vi "Opt2.vi"(0 "Activation Function":enum32{"Sigmoid", "RELU", "Tanh", "Leaky RELU"}(ring), 1 "Weights l+1":dbl[](array[numeric]), 2 "Weights":dbl[][](array[numeric]), 3 "Biases":dbl[](array[numeric]), 5 "Net Output":dbl[](array[numeric]), 7 "Activations l-1":dbl[](array[numeric]) format="%.2f", 9 "Delta l+1":dbl, 12 "Weight Regularizers":enum32{"None", "L1", "L2"}(radio), 13 "Adam Data In":T1) -> (4 "Delta l":dbl[](array[numeric]), 6 "Updated Weights":dbl[][](array[numeric]), 8 "Updated Biases":dbl[](array[numeric]), 14 "Adam Data Out":T1)   [LabVIEW 2018]
uses:
  Adam_data.ctl
  <vilib>/Analysis/baseanly.llb/Real Outer Product.vi
  <vilib>/Analysis/Matrix/Numeric/Conversions/Matrix To Array - RM.vi
  Iteration Counter.vi
  <vilib>/Analysis/NI_AALBase.lvlib
  <vilib>/Analysis/Matrix/NI_Matrix.lvlib
panel:
  out "Grad. w":dbl[][](array[numeric])
  out "Grad. b":dbl[](array[numeric])
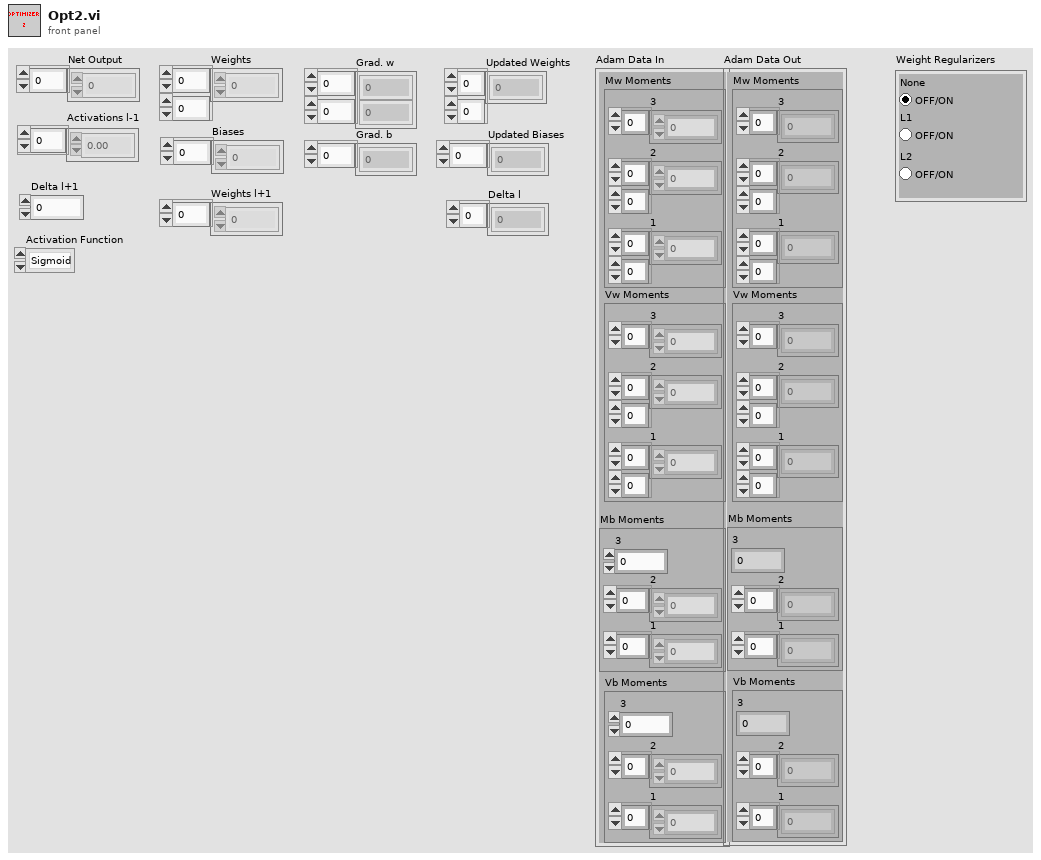
[diagram p1: front panel]
types:
  T1 = typedef "Adam_data.ctl" = cluster{"Mw Moments":cluster{"3 ":dbl[], "2":dbl[][], "1":dbl[][]}, "Vw Moments":cluster{"3":dbl[], "2":dbl[][], "1":dbl[][]}, "Mb Moments":cluster{"3":dbl, "2":dbl[], "1":dbl[]}, "Vb Moments":cluster{"3":dbl, "2":dbl[], "1":dbl[]}}
  T2 = typedef "NI_Matrix.lvlib/RealMatrix.ctl" = dbl[][]
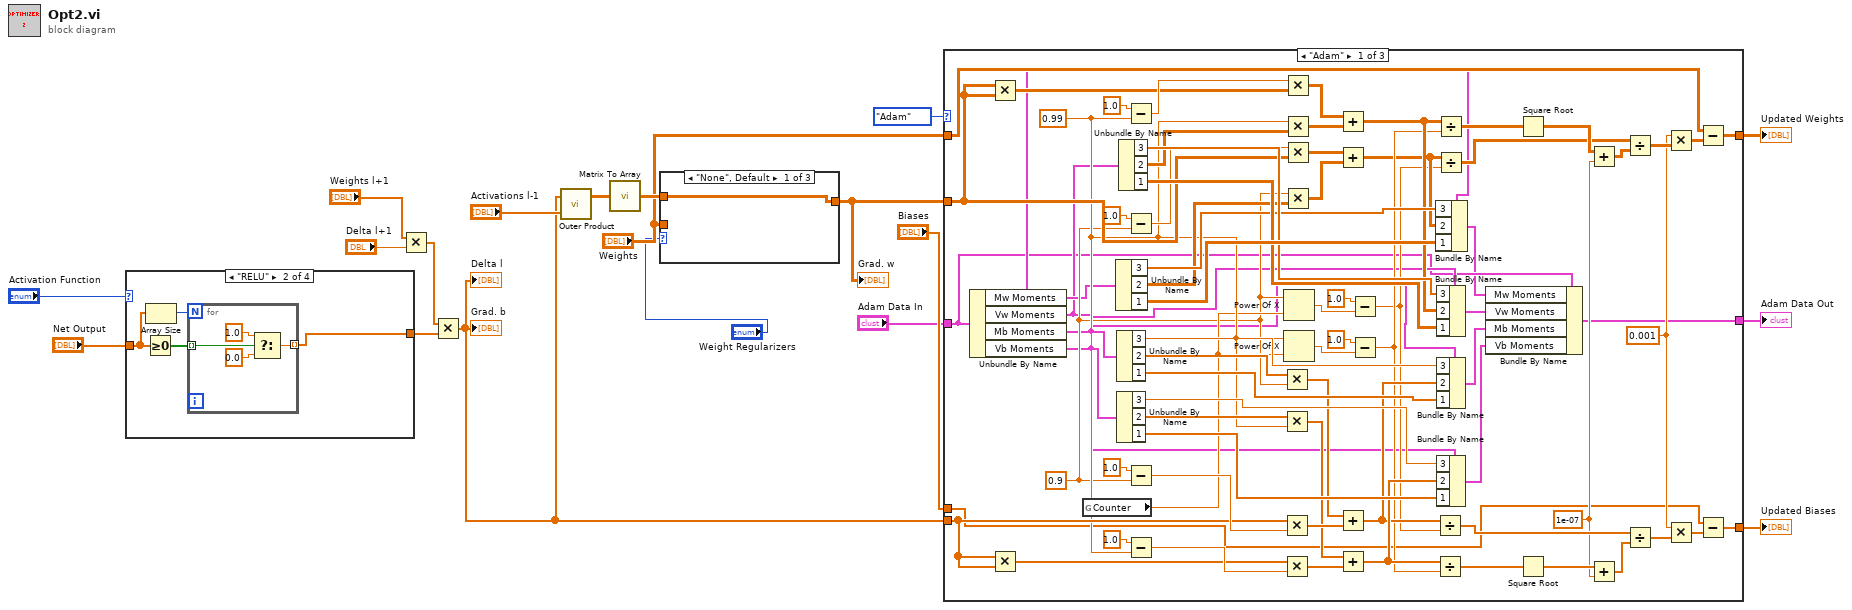
[diagram p0: block diagram]
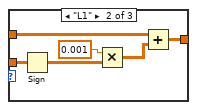
[diagram p2: hidden frame]
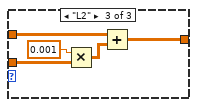
[diagram p3: hidden frame]
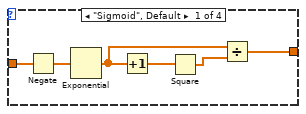
[diagram p6: hidden frame]
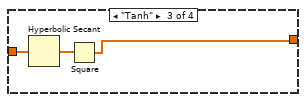
[diagram p7: hidden frame]
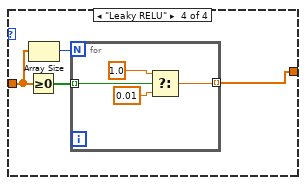
[diagram p8: hidden frame]
diagram:
  n1 = case shown="\"RELU\"" "Activation Function" {
    tunnel: "Net Output" -> [w21 w27 w35 w38]
    tunnel: [w20 w29 w34 w40] -> w18
    frame "Sigmoid", Default {
      n2 = Negate(x=w21) -> (-x=w25:dbl[])
      n3 = Exponential(1:w25) -> (0:w22:dbl[])
      n4 = Increment(x=w22) -> (x+1=w24:dbl[])
      n5 = Square(x=w24) -> (x^2=w23:dbl[])
      n6 = Divide(x=w22, y=w23) -> (x/y=w20:dbl[])
    }
    frame "RELU" {
      n7 = Greater Or Equal To 0?(x=w27) -> (x >= 0?=w28:bool[])
      n8 = Array Size(array=w27) -> (size(s)=w26:i32)
      n9 = for {
        N: w26 -> [_]
        tunnel: [w33] -> w29 mode=indexing
        tunnel: w28 -> [w30] mode=indexing
        n10 = Select(t=1.0, s=w30, f=0.0) -> (s? t:f=w33:dbl)
      }
    }
    frame "Tanh" {
      n11 = Hyperbolic Secant(1:w35) -> (0:w36:dbl[])
      n12 = Square(x=w36) -> (x^2=w34:dbl[])
    }
    frame "Leaky RELU" {
      n13 = Greater Or Equal To 0?(x=w38) -> (x >= 0?=w39:bool[])
      n14 = Array Size(array=w38) -> (size(s)=w37:i32)
      n15 = for {
        N: w37 -> [_]
        tunnel: [w42] -> w40 mode=indexing
        tunnel: w39 -> [w41] mode=indexing
        n16 = Select(t=1.0, s=w41, f=0.01) -> (s? t:f=w42:dbl)
      }
    }
  }
  n17 = Multiply(x="Weights l+1", y="Delta l+1") -> (x*y=w8:dbl[])
  n18 = Multiply(x=w8, y=w18) -> (x*y=w14:dbl[])
  "Grad. b" <- w14
  "Delta l" <- w14
  n19 = call-poly <vilib>:"Outer Product.vi"("Y Vector"="Activations l-1", "X Vector"=w14) -> ("Outer Product"=w13:T2)  [unwired: 1 out]
  n20 = call-poly <vilib>:"Matrix To Array.vi"("Real Matrix"=w13) -> ("Real 2D Array"=w4:dbl[][])
  n21 = case shown="\"None\", Default" "Weight Regularizers" {
    tunnel: w4 -> [w45 w47 w56]
    tunnel: [w45 w46 w52] -> w2
    tunnel: "Weights" -> [_ w50 w54]
    frame "None", Default {
    }
    frame "L1" {
      n22 = Sign(1:w50) -> (0:w49:dbl[][])
      n23 = Multiply(x=0.001, y=w49) -> (x*y=w48:dbl[][])
      n24 = Add(x=w47, y=w48) -> (x+y=w46:dbl[][])
    }
    frame "L2" {
      n25 = Multiply(x=0.001, y=w54) -> (x*y=w53:dbl[][])
      n26 = Add(x=w56, y=w53) -> (x+y=w52:dbl[][])
    }
  }
  "Grad. w" <- w2
  n27 = case shown="\"Adam\"" enum16{"Adagrad", "Adadelta", "Adam"}."Adam" ("Optimizer") {
    tunnel: "Weights" -> [w68 w132 w135]
    tunnel: [w67 w132 w135] -> w12
    tunnel: "Biases" -> [w71 w131 w134]
    tunnel: [w70 w131 w134] -> w16
    tunnel: w14 -> [w115 _ _]
    tunnel: w2 -> [w100 _ _]
    tunnel: "Adam Data In" -> [w62 w130 w133]
    tunnel: [w57 w130 w133] -> w6
    frame "Adam" {
      w77 = 1e-07
      w73 = 0.001
      w97 = 0.99
      w92 = 0.9
      n28 = Unbundle By Name(w62) -> ("Mw Moments"=w64:cluster{"3 ":dbl[], "2":dbl[][], "1":dbl[][]}, "Vw Moments"=w63:cluster{"3":dbl[], "2":dbl[][], "1":dbl[][]}, "Mb Moments"=w66:cluster{"3":dbl, "2":dbl[], "1":dbl[]}, "Vb Moments"=w65:cluster{"3":dbl, "2":dbl[], "1":dbl[]})
      n29 = Multiply(x=w100, y=w100) -> (x*y=w104:dbl[][])
      n30 = Multiply(x=w115, y=w115) -> (x*y=w114:dbl[])
      n31 = global read "Iteration Counter.vi" "Counter"() -> (w93:dbl)
      n32 = Unbundle By Name(w64) -> ("3"=w110:dbl[], "2"=w103:dbl[][], "1"=w129:dbl[][])
      n33 = Unbundle By Name(w66) -> ("3"=w124:dbl, "2"=w123:dbl[], "1"=w127:dbl[])
      n34 = Unbundle By Name(w65) -> ("3"=w125:dbl, "2"=w118:dbl[], "1"=w126:dbl[])
      n35 = Unbundle By Name(w63) -> ("3"=w111:dbl[], "2"=w109:dbl[][], "1"=w128:dbl[][])
      n36 = Subtract(x=1.0, y=w97) -> (x-y=w107:dbl)
      n37 = Subtract(x=1.0, y=w92) -> (x-y=w101:dbl)
      n38 = Subtract(x=1.0, y=w92) -> (x-y=w121:dbl)
      n39 = Subtract(x=1.0, y=w97) -> (x-y=w116:dbl)
      n40 = Multiply(x=w123, y=w92) -> (x*y=w120:dbl[])
      n41 = Multiply(x=w118, y=w97) -> (x*y=w113:dbl[])
      n42 = Multiply(x=w115, y=w121) -> (x*y=w119:dbl[])
      n43 = Multiply(x=w114, y=w116) -> (x*y=w112:dbl[])
      n44 = Multiply ("Multiply.vi")(x=w107, y=w104) -> (x*y=w106:dbl[][])
      n45 = Multiply(x=w97, y=w109) -> (x*y=w105:dbl[][])
      n46 = Multiply(x=w101, y=w100) -> (x*y=w99:dbl[][])
      n47 = Multiply(x=w92, y=w103) -> (x*y=w98:dbl[][])
      n48 = Power Of X(1:w93, 2:w92) -> (0:w90:dbl)
      n49 = Power Of X(1:w93, 2:w97) -> (0:w96:dbl)
      n50 = Add(x=w106, y=w105) -> (x+y=w88:dbl[][])
      n51 = Add(x=w99, y=w98) -> (x+y=w86:dbl[][])
      n52 = Add(x=w120, y=w119) -> (x+y=w89:dbl[])
      n53 = Add(x=w113, y=w112) -> (x+y=w94:dbl[])
      n54 = Subtract(x=1.0, y=w90) -> (x-y=w85:dbl)
      n55 = Subtract(x=1.0, y=w96) -> (x-y=w87:dbl)
      n56 = Divide(x=w89, y=w85) -> (x/y=w81:dbl[])
      n57 = Divide(x=w94, y=w87) -> (x/y=w84:dbl[])
      n58 = Divide(x=w88, y=w87) -> (x/y=w79:dbl[][])
      n59 = Divide(x=w86, y=w85) -> (x/y=w76:dbl[][])
      n60 = Bundle By Name(cluster=w64, "3"=w110, "2"=w86, "1"=w129) -> (w61:cluster{"3 ":dbl[], "2":dbl[][], "1":dbl[][]})
      n61 = Bundle By Name(cluster=w63, "3"=w111, "2"=w88, "1"=w128) -> (w60:cluster{"3":dbl[], "2":dbl[][], "1":dbl[][]})
      n62 = Bundle By Name(cluster=w66, "3"=w124, "2"=w89, "1"=w127) -> (w59:cluster{"3":dbl, "2":dbl[], "1":dbl[]})
      n63 = Bundle By Name(cluster=w65, "3"=w125, "2"=w94, "1"=w126) -> (w58:cluster{"3":dbl, "2":dbl[], "1":dbl[]})
      n64 = Bundle By Name(cluster=w62, "Mw Moments"=w61, "Vw Moments"=w60, "Mb Moments"=w59, "Vb Moments"=w58) -> (w57:T1)
      n65 = Square Root(x=w79) -> (sqrt(x)=w78:dbl[][])
      n66 = Square Root(x=w84) -> (sqrt(x)=w83:dbl[])
      n67 = Add(x=w78, y=w77) -> (x+y=w75:dbl[][])
      n68 = Add(x=w83, y=w77) -> (x+y=w82:dbl[])
      n69 = Divide(x=w76, y=w75) -> (x/y=w74:dbl[][])
      n70 = Divide(x=w81, y=w82) -> (x/y=w80:dbl[])
      n71 = Multiply(x=w73, y=w74) -> (x*y=w69:dbl[][])
      n72 = Multiply(x=w73, y=w80) -> (x*y=w72:dbl[])
      n73 = Subtract(x=w68, y=w69) -> (x-y=w67:dbl[][])
      n74 = Subtract(x=w71, y=w72) -> (x-y=w70:dbl[])
    }
    frame "Adadelta" {
    }
    frame "Adagrad" {
    }
  }
  "Updated Biases" <- w16
  "Updated Weights" <- w12
  "Adam Data Out" <- w6
